vi "Save Settings.vi"(8 "error in (no error)":errorcluster {"code" format="Error %.0f"}, 11 "Printer Settings In":refnum<class "Printer Settings.lvclass">) -> (0 "error out":errorcluster {"code" format="Error %.0f"}, 3 "Printer Settings Out":refnum<class "Printer Settings.lvclass">)   [LabVIEW 2023, in "VIDoc Printer.lvlib" / "Printer Settings.lvclass"]
uses:
  Printer Settings.lvclass
  C:/projects/DMC/Tooling/Git-Action-Service/Source/Documentation Generation/Settings/VIDoc Settings/VIDoc Settings.lvclass
  Printer Settings.lvclass/Printer Settings.ctl
  VIDoc Settings/VIDoc Settings.lvclass/VIDoc Settings.ctl
  VIDoc Settings/Get VIDoc Settings Path.vi
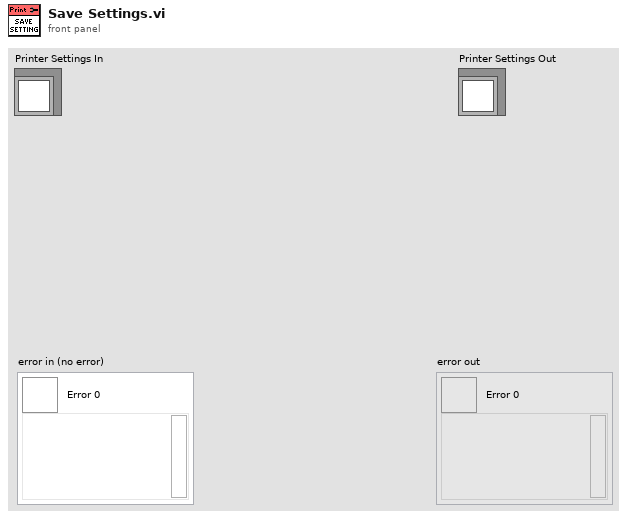
[diagram p1: front panel]
types:
  T1 = typedef "VIDoc Printer.lvlib/Printer Settings.lvclass/Enabled Sections Cluster.ctl" = cluster{"Projects":bool, "User Interfaces":bool, "Subpanels":bool, "Dialogs":bool, "Interfaces":bool, "Classes":bool, "Libraries":bool, "VIs":bool, "Controls":bool, "LLBs":bool}
  T2 = typedef "VIDoc Printer.lvlib/Printer Settings.lvclass/Printer Settings Cluster.ctl" = cluster{"Project":T3, "User Interface":T4, "Subpanel":T4, "Dialog":T4, "VI Member":T4, "Interface":T6, "Class":T8, "Library":T9, "Control Member":T10, "Format Options":T11, "Library Scope":cluster{"Public":bool, "Community":bool, "Private":bool, "Unknown":bool}, "LLB":T14}
  T3 = typedef "VIDoc Printer.lvlib/Printer Settings.lvclass/Project Settings.ctl" = cluster{"Paths":bool, "Descriptions":bool, "Memory":bool, "Options":bool, "Symbols":bool}
  T4 = typedef "VIDoc Printer.lvlib/Printer Settings.lvclass/VI Settings.ctl" = cluster{"Memory":bool, "By Folder":bool, "By Tree":bool, "By List":bool, "Methods":bool, "Method Options":cluster{"Front Panels":bool, "Options":bool, "Controls":bool}, "List Detail Level":T5, "Methods Detail Level":T5, "Controls Detail Level":T5}
  T5 = typedef "VIDoc Printer.lvlib/Printer Settings.lvclass/Detail Level Enum.ctl" = enum16{"None", "Minimal", "Standard", "Full"}
  T6 = typedef "VIDoc Printer.lvlib/Printer Settings.lvclass/Interface Settings.ctl" = cluster{"Memory":bool, "By List":bool, "Details":bool, "Detail Options":cluster{"Description":bool, "Properties":bool, "Inheritance":bool, "Inheritance Options":cluster{"Parent Interfaces":bool, "Friends":bool}}, "List Detail Level":T5, "Controls Detail Level":T5, "Methods Detail Level":T5, "Controls Scope":T7, "Methods Scope":T7}
  T7 = typedef "VIDoc Printer.lvlib/Printer Settings.lvclass/Scope Settings.ctl" = cluster{"Public":bool, "Protected":bool, "Community":bool, "Private":bool, "Unknown":bool}
  T8 = typedef "VIDoc Printer.lvlib/Printer Settings.lvclass/Class Settings.ctl" = cluster{"Memory":bool, "By Folder":bool, "By Tree":bool, "By List":bool, "Details":bool, "Detail Options":cluster{"Description":bool, "Properties":bool, "Inheritance":bool, "Inheritance Options":cluster{"Parent Classes":bool, "Parent Interfaces":bool, "Parent Libraries":bool, "Friends":bool}}, "CPD Detail Level":T5, "List Detail Level":T5, "Controls Detail Level":T5, "Methods Detail Level":T5, "Set Accessor Detail Level":T5, "Get Accessor Detail Level":T5, "Controls Scope":T7, "Methods Scope":T7, "Get Accessors Scope":T7, "Set Accessors Scope":T7}
  T9 = typedef "VIDoc Printer.lvlib/Printer Settings.lvclass/Library Settings.ctl" = cluster{"Memory":bool, "By Folder":bool, "By Tree":bool, "By List":bool, "Details":bool, "Detail Options":cluster{"Description":bool, "Properties":bool, "Friends":bool, "Child Libraries":bool}, "List Detail Level":T5, "Methods Detail Level":T5, "Controls Detail Level":T5, "Methods Scope":T7, "Controls Scope":T7}
  T10 = typedef "VIDoc Printer.lvlib/Printer Settings.lvclass/Control Settings.ctl" = cluster{"Memory":bool, "By Folder":bool, "By Tree":bool, "By List":bool, "Controls":bool, "List Detail Level":T5, "Controls Detail Level":T5}
  T11 = typedef "VIDoc Printer.lvlib/Printer Settings.lvclass/Formatting Options.ctl" = cluster{"Background":cluster{"Public Scope":T12, "Protected Scope":T12, "Community Scope":T12, "Private Scope":T12, "Unknown Scope":T12, "Auto Error Handling":T12, "Inline":T12, "Separate CC":T12, "Execution Priority Normal":T12, "Reentrancy Non-RE":T12}, "Bookmark Options":T13}
  T12 = typedef "VIDoc Printer.lvlib/Printer Settings.lvclass/Background Formatting Cluster.ctl" = cluster{"Option":bool, "Color":u32, "Operator":bool}
  T13 = typedef "VIDoc Printer.lvlib/Printer Settings.lvclass/Bookmark Options.ctl" = cluster{"Bookmarks as New Line in VI Descriptions":bool, "Unique Bookmark Tags Only":bool, "Include Tag and Text":bool}
  T14 = typedef "VIDoc Printer.lvlib/Printer Settings.lvclass/LLB Settings.ctl" = cluster{"Methods":bool, "Controls":bool, "Methods Detail Level":T5, "Controls Detail Level":T5}
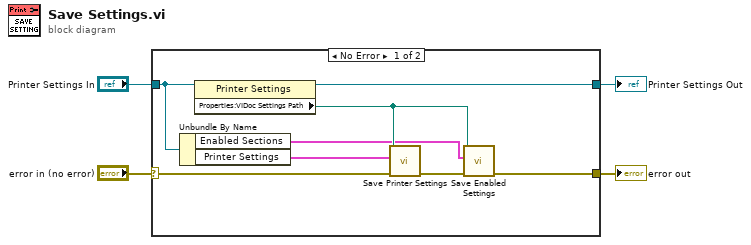
[diagram p0: block diagram]
diagram:
  n1 = case shown="No Error" "error in (no error)" {
    selector: "error in (no error)" -> [w10 w13]
    tunnel: [w8 w13] -> w4
    tunnel: [w12 w14] -> w2
    tunnel: "Printer Settings In" -> [w11 w14]
    frame No Error {
      n2 = Unbundle By Name(w11) -> ("Enabled Sections"=w5:T1, "Printer Settings"=w6:T2)
      n3 = property class="Printer Settings"(reference=w11) -> (reference out=w12:refnum<class "Printer Settings.lvclass">, "Properties:VIDoc Settings Path"=w7:path)  [unwired: 1 in, 1 out]
      n4 = call "Save Printer Settings.vi"("Error in"=w10, "Printer Settings"=w6, "Settings Path"=w7) -> ("Error out"=w9:errorcluster)  [unwired: 8 in]
      n5 = call "Save Enabled Settings.vi"("Error in"=w9, "Enabled Sections"=w5, "Settings Path"=w7) -> ("Error out"=w8:errorcluster)  [unwired: 8 in]
    }
    frame Error {
    }
  }
  "error out" <- w4
  "Printer Settings Out" <- w2
